vi "Charger_Multi-Channel Setup.vi"(6 "STOP Refnum":refnum<vi>, 7 "Status Refnum  Array":T1[](array[typedef]), 8 "error in":errorcluster) -> (0 "error out":errorcluster)   [LabVIEW 2020]
doc: "This function performs the preliminary setup for all IPGs that are ready to charge, waits 13 seconds for IPG startup (displays stopwatch), then completes the remaining setup (open IPG session and starts IPG charging)."
uses:
  Charger_Status Refnum.ctl
  Drivers/Charger Test Set/Charger_Input Control.ctl
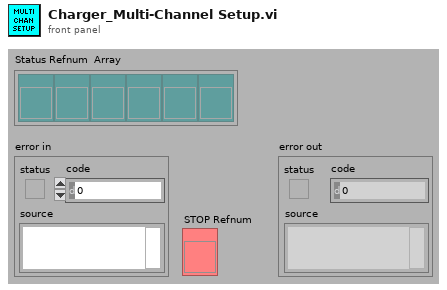
[diagram p1: front panel]
types:
  T1 = typedef "Charger_Status Refnum.ctl" = refnum<vi>
  T2 = typedef "MICS_Input Control.ctl" = cluster{"address":refnum<visa-resource-name>, "chan":u16, "ID":u32}
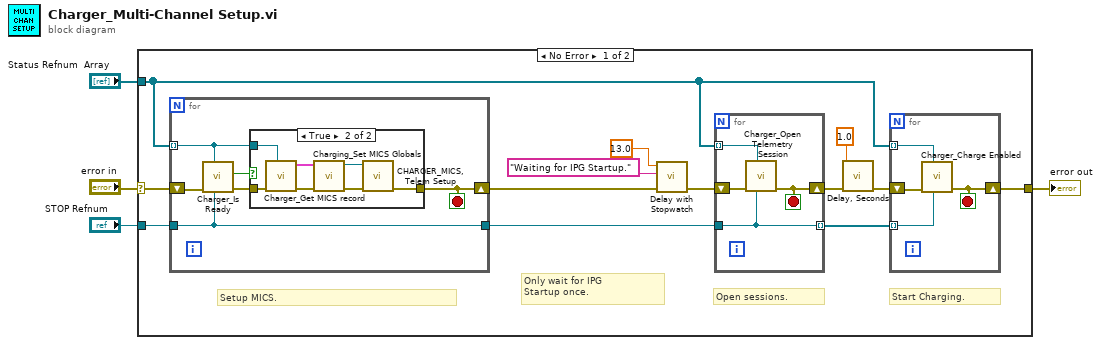
[diagram p0: block diagram]
diagram:
  n1 = case shown="No Error" "error in" {
    selector: "error in" -> [w13 w40]
    tunnel: [w5 w40] -> w2
    tunnel: "Status Refnum  Array" -> [w6 _]
    tunnel: "STOP Refnum" -> [w17 _]
    frame No Error {
      # "Start Charging."
      # "Open sessions."
      # "Setup MICS."
      # "Only wait for IPG\nStartup once."
      n2 = for {
        tunnel: w17 -> [w31]
        shift-right: [w30] -> w15
        shift-left: w13 -> [w26]
        tunnel: w6 -> [w27] mode=indexing
        tunnel: [w31] -> w16
        stop <- w30 stop-if-true
        n3 = call "Charger_Is Ready.vi"("Stop Refnum"=w31, "Status Refnum"=w27, "error in"=w26) -> ("error out"=w29:errorcluster, "ready"=w28:bool)  [unwired: 7 in]
        n4 = case shown="True" w28 {
          tunnel: [w32 w39] -> w30
          tunnel: w29 -> [w32 w36]
          tunnel: w27 -> [_ w33]
          frame False {
          }
          frame True {
            n5 = call "Charger_Get MICS record.vi"("Status Refnum"=w33, "error in"=w36) -> ("error out"=w35:errorcluster, "MICS Inputs"=w34:T2)  [unwired: 3 in, 3 out]
            n6 = call "Charging_Set MICS Globals.vi"("error in"=w35, "MICS inputs"=w34) -> ("error out"=w37:errorcluster, "address"=w38:refnum<visa-resource-name>)  [unwired: 4 in]
            n7 = call "CHARGER_MICS, Telem Setup.vi"("error in"=w37, "VISA resource"=w38) -> ("error out"=w39:errorcluster)  [unwired: 8 in, 1 out]
          }
        }
      }
      n8 = call "Delay with Stopwatch.vi"("error in"=w15, "window title"="Waiting for IPG Startup.", "delay"=dbl[unit] 13.0 ("Startup Delay (13 s)")) -> ("error out"=w14:errorcluster)  [unwired: 4 in]
      n9 = for {
        tunnel: w16 -> [w22]
        shift-right: [w23] -> w9
        shift-left: w14 -> [w24]
        tunnel: w6 -> [w25] mode=indexing
        tunnel: [w22] -> w7 mode=indexing
        stop <- w23 stop-if-true
        n10 = call "Charger_Open Telemetry Session.vi"("Stop Refnum"=w22, "Status Refnum"=w25, "error in"=w24) -> ("error out"=w23:errorcluster)  [unwired: 7 in, 1 out]
      }
      n11 = call "Delay, Seconds.vi"("error in"=w9, "delay"=dbl[unit] 1.0) -> ("error out"=w8:errorcluster)  [unwired: 5 in, 1 out]
      n12 = for {
        shift-right: [w18] -> w5
        shift-left: w8 -> [w19]
        tunnel: w7 -> [w21] mode=indexing
        tunnel: w6 -> [w20] mode=indexing
        stop <- w18 stop-if-true
        n13 = call "Charger_Charge Enabled.vi"("Stop Refnum"=w21, "Status Refnum"=w20, "error in"=w19) -> ("error out"=w18:errorcluster)  [unwired: 8 in]
      }
    }
    frame Error {
    }
  }
  "error out" <- w2
